vi "HDF5_WriteComplexSpectrums.vi"(8 "error in":errorcluster, 10 "ToneData":T1={"Count"=0, "CalVal"=[], "CalLoc"=[], "BeacVal"=[], "BeacLoc"=[], "BeacShift"=[], "Enum"=enum."4", "df"=0.0, "PwrSpectr"=[], "ISpectr"=[], "QSpectr"=[], "Time"=[], "SNR"=[], "AboveThresh"=[], "10Hz_PeakVal"=[], "Phase"=[], "DeltaPhase"=[], "Saturat"={"Meas"=[], "Stage1"=[], "Stage4"=[], "Stage5"=[], "Stage6"=[], "Stage7"=[]}, "10MHz"=FALSE}, 11 "Complex Refs":T4 {"Group_ref" format="%.0x"; "QSpect_dset" format="%.0x"; "ISpect_dset" format="%.0x"; "PwrSpect_dset" format="%.0x"; "TImeStamp_dset" format="%.0x"}) -> (0 "error out":errorcluster)   [LabVIEW 2018]
uses:
  HDF5_Complex_Refs.ctl
  <vilib>/addons/h5labview2/base/hid_t.ctl
  Controls/Clusts/ToneLogBuffered.ctl
  Controls/Enums/TargetNumber.ctl
  Controls/Clusts/SaturationMonitorBuffer.ctl
  <vilib>/addons/h5labview2/base/H5Equery.vi
  <vilib>/addons/h5labview2/dataset/H5Dwrite.llb/H5Dwrite.xnode
  <vilib>/addons/h5labview2/space/H5S.lvlib
  <vilib>/addons/h5labview2/dataset/H5D.lvlib
  <vilib>/addons/h5labview2/base/lib_path.vi
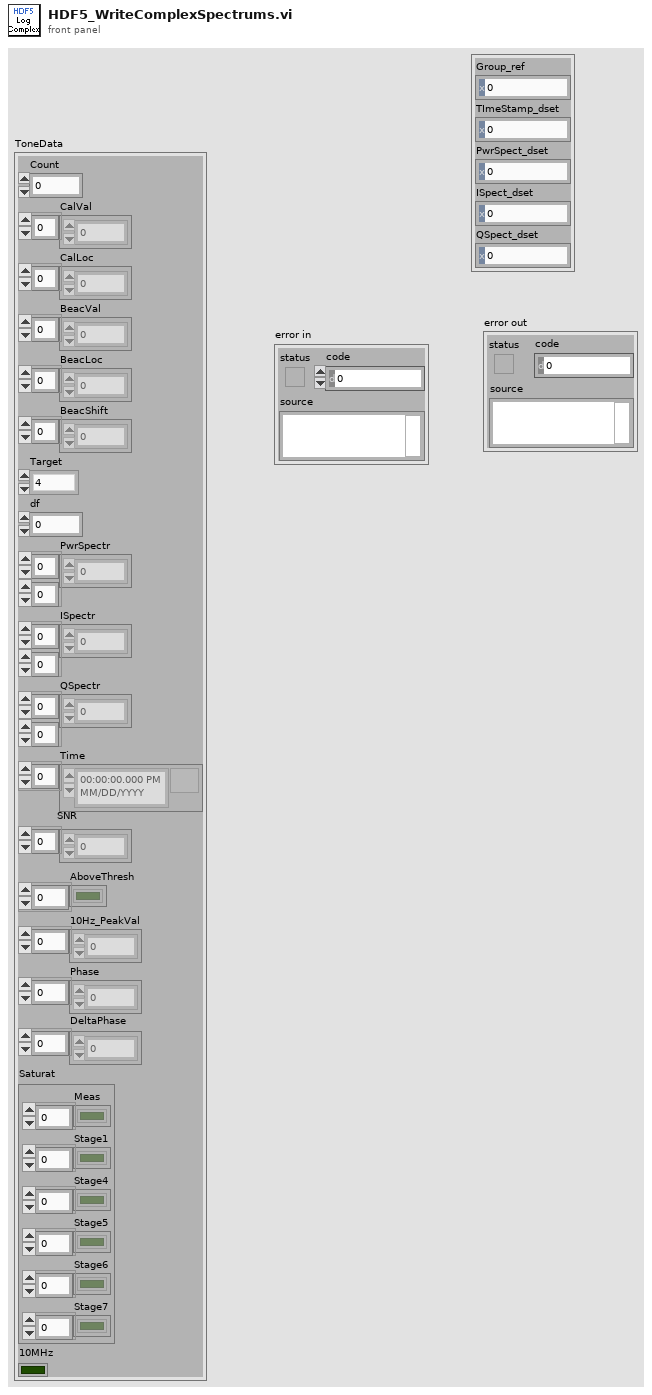
[diagram p1: front panel]
types:
  T1 = typedef "ToneLogBuffered.ctl" = cluster{"Count":i32, "CalVal":sgl[], "CalLoc":i32[], "BeacVal":sgl[], "BeacLoc":i32[], "BeacShift":i32[], "Enum":T2, "df":dbl, "PwrSpectr":sgl[][], "ISpectr":sgl[][], "QSpectr":sgl[][], "Time":timestamp[], "SNR":sgl[], "AboveThresh":bool[], "10Hz_PeakVal":dbl[], "Phase":sgl[], "DeltaPhase":dbl[], "Saturat":T3, "10MHz":bool}
  T2 = typedef "TargetNumber.ctl" = enum16{"1", "2", "3", "4"}
  T3 = typedef "SaturationMonitorBuffer.ctl" = cluster{"Meas":bool[], "Stage1":bool[], "Stage4":bool[], "Stage5":bool[], "Stage6":bool[], "Stage7":bool[]}
  T4 = typedef "HDF5_Complex_Refs.ctl" = cluster{"Group_ref":T5, "TImeStamp_dset":T5, "PwrSpect_dset":T5, "ISpect_dset":T5, "QSpect_dset":T5}
  T5 = typedef "hid_t.ctl" = i32
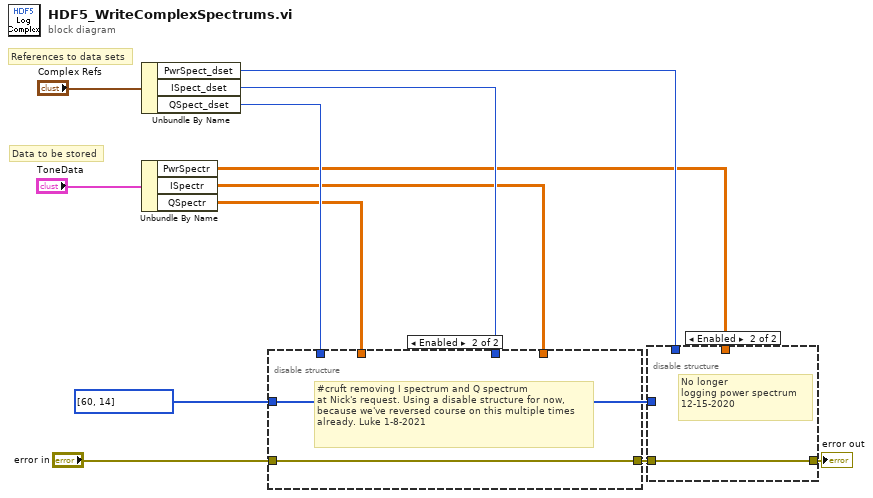
[diagram p0: block diagram]
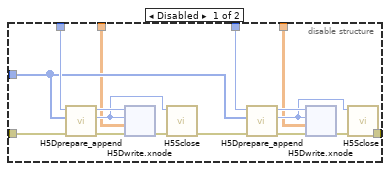
[diagram p2: hidden frame]
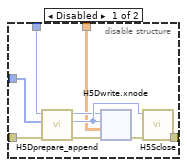
[diagram p3: hidden frame]
diagram:
  w4 = u64[] [60, 14] ("append dims")
  # "References to data sets"
  # "Data to be stored"
  n1 = Unbundle By Name("Complex Refs") -> ("PwrSpect_dset"=w11:T5, "ISpect_dset"=w12:T5, "QSpect_dset"=w5:T5)
  n2 = Unbundle By Name("ToneData") -> ("PwrSpectr"=w3:sgl[][], "ISpectr"=w2:sgl[][], "QSpectr"=w1:sgl[][])
  n3 = disable-structure shown="Enabled" {
    disable-tunnel: w12 -> [w28 _]
    disable-tunnel: [w27 w67] -> w10
    disable-tunnel: "error in" -> [w18 w67]
    disable-tunnel: w5 -> [w17 _]
    disable-tunnel: w4 -> [w16 _]
    disable-tunnel: w2 -> [w14 _]
    disable-tunnel: w1 -> [w13 _]
    frame Disabled {
      n4 = call <vilib>:"H5Dprepare_append.vi"("error in (no error)"=w18, "append dims"=w16, "dset in"=w17) -> ("error out"=w21:errorcluster, "space out"=w15:T5, "dset out"=w22:T5)  [unwired: 5 in, 1 out]
      n5 = xnode "H5Dwrite.xnode"("error in (no error)"=w21, "data"=w13, "file space"=w15, "ref in"=w22) -> ("error out"=w20:errorcluster)  [unwired: 3 in, 2 out]
      n6 = call <vilib>:"H5Sclose.vi"("error in (no error)"=w20, "space in"=w15) -> ("error out"=w19:errorcluster)  [unwired: 9 in]
      n7 = call <vilib>:"H5Dprepare_append.vi"("error in (no error)"=w19, "append dims"=w16, "dset in"=w28) -> ("error out"=w25:errorcluster, "space out"=w23:T5, "dset out"=w24:T5)  [unwired: 5 in, 1 out]
      n8 = xnode "H5Dwrite.xnode"("error in (no error)"=w25, "data"=w14, "file space"=w23, "ref in"=w24) -> ("error out"=w26:errorcluster)  [unwired: 3 in, 2 out]
      n9 = call <vilib>:"H5Sclose.vi"("error in (no error)"=w26, "space in"=w23) -> ("error out"=w27:errorcluster)  [unwired: 9 in]
    }
    frame Enabled {
      # "#cruft removing I spectrum and Q spectrum\nat Nick's request. Using a disable structure for now,\nbecause we've reversed course on this multiple times already. Luke 1-8-2021"
    }
  }
  n10 = disable-structure shown="Enabled" {
    disable-tunnel: w11 -> [w76 _]
    disable-tunnel: w10 -> [w75 w96]
    disable-tunnel: [w70 w96] -> w8
    disable-tunnel: w4 -> [w69 _]
    disable-tunnel: w3 -> [w68 _]
    frame Disabled {
      n11 = call <vilib>:"H5Dprepare_append.vi"("error in (no error)"=w75, "append dims"=w69, "dset in"=w76) -> ("error out"=w72:errorcluster, "space out"=w74:T5, "dset out"=w73:T5)  [unwired: 5 in, 1 out]
      n12 = xnode "H5Dwrite.xnode"("error in (no error)"=w72, "data"=w68, "file space"=w74, "ref in"=w73) -> ("error out"=w71:errorcluster)  [unwired: 3 in, 2 out]
      n13 = call <vilib>:"H5Sclose.vi"("error in (no error)"=w71, "space in"=w74) -> ("error out"=w70:errorcluster)  [unwired: 9 in]
    }
    frame Enabled {
      # "No longer\nlogging power spectrum\n12-15-2020"
    }
  }
  "error out" <- w8
